vi "Kenimatics_Translation2d_ADD.vi"(9 "Other Translation":T1 {"Y" format="%14.3f"; "X" format="%14.3f"}, 11 "In Translation":T1 {"Y" format="%14.3f"; "X" format="%14.3f"}) -> (3 "Out Translation Out":T1 {"Y" format="%14.3f"; "X" format="%14.3f"})   [LabVIEW 2023, in "Swerve_Odometry_SEN.lvlib"]
doc: "Adds two translations in 2d space and returns the sum. This is similar to vector addition.\n \nFor example, Translation2d{1.0, 2.5} + Translation2d{2.0, 5.5} = Translation2d{3.0, 8.0}\n\nParameters:\n - IN Translation - This translation data structure\n - other Translation - The translation data structure to add\n\nReturns\n - Out Translation - The summation of the two translations."
uses:
  Swerve_Odometry_SEN.lvlib
  Cluster_TRANSLATION2D.ctl
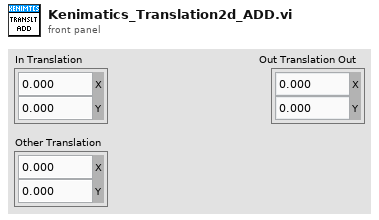
[diagram p1: front panel]
types:
  T1 = typedef "Swerve_Odometry_SEN.lvlib/Cluster_TRANSLATION2D.ctl" = cluster{"X":dbl, "Y":dbl}
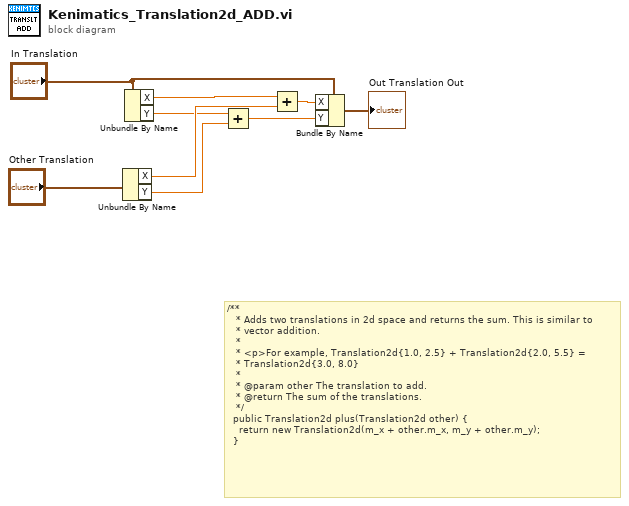
[diagram p0: block diagram]
diagram:
  # "/**\n   * Adds two translations in 2d space and returns the sum. This is similar to\n   * vector addition.\n   *\n   * <p>For example, Translation2d{1.0, 2.5} + Translation2d{2.0, 5.5} =\n   * Translation2d{3.0, 8.0}\n   *\n   * @param other The translation to add.\n   * @return The sum of the translations.\n   */\n  public Translation2d plus(Translation2d other) {\n    return new Translation2d(m_x + other.m_x, m_y + other.m_y);\n  }"
  n1 = Unbundle By Name("Other Translation") -> ("X"=w7:dbl, "Y"=w6:dbl)
  n2 = Unbundle By Name("In Translation") -> ("X"=w8:dbl, "Y"=w5:dbl)
  n3 = Add(x=w5, y=w6) -> (x+y=w1:dbl)
  n4 = Add(x=w8, y=w7) -> (x+y=w2:dbl)
  n5 = Bundle By Name(cluster="In Translation", "X"=w2, "Y"=w1) -> (→"Out Translation Out":T1)
